vi "未命名 3.vi"() -> ()   [LabVIEW 2018]
panel:
  in  "数值":dbl
  out "簇 2":cluster{"数值":dbl, "数值 2":dbl}
  in  "簇":cluster{"数值":dbl, "数值 2":dbl}
  out "数组 3":i32[][](array[numeric])
  out "添加的数组":dbl[](array[numeric])
  out "数组 2":i32[](array[numeric])
  in  "数组":dbl[](array[numeric])
  out "波形图 2":dynamicdata(graph)
  out "波形图":dynamicdata(graph)
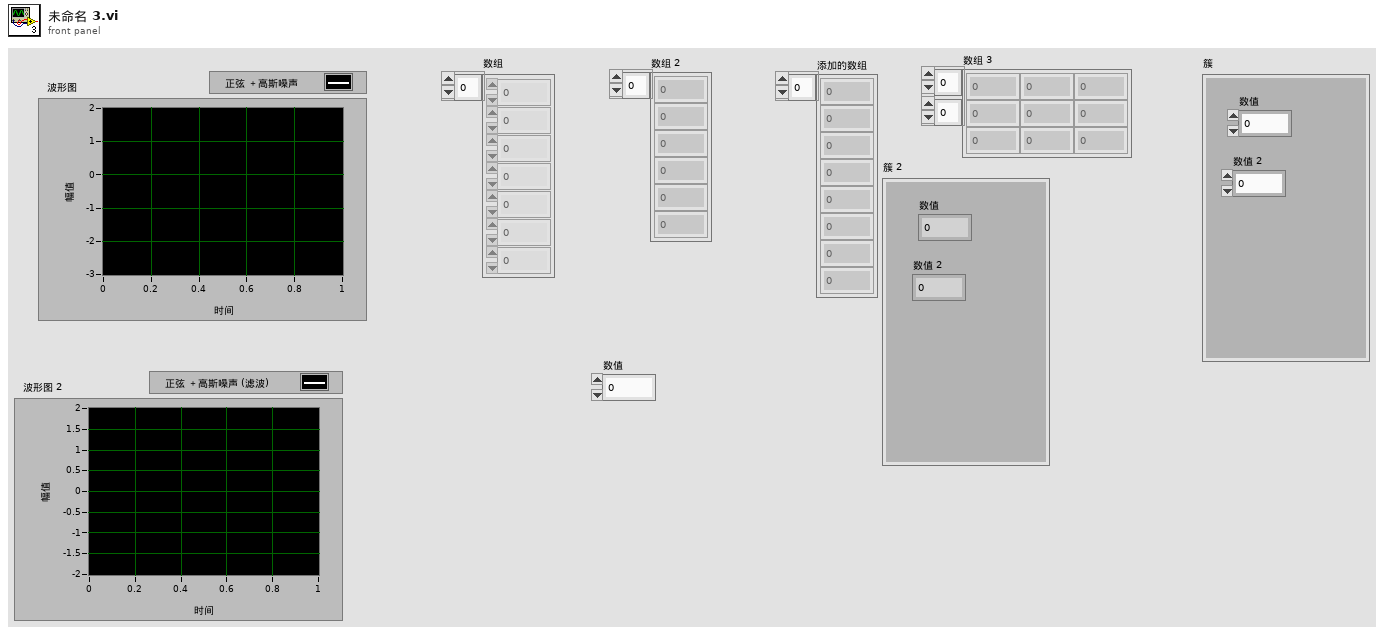
[diagram p1: front panel]
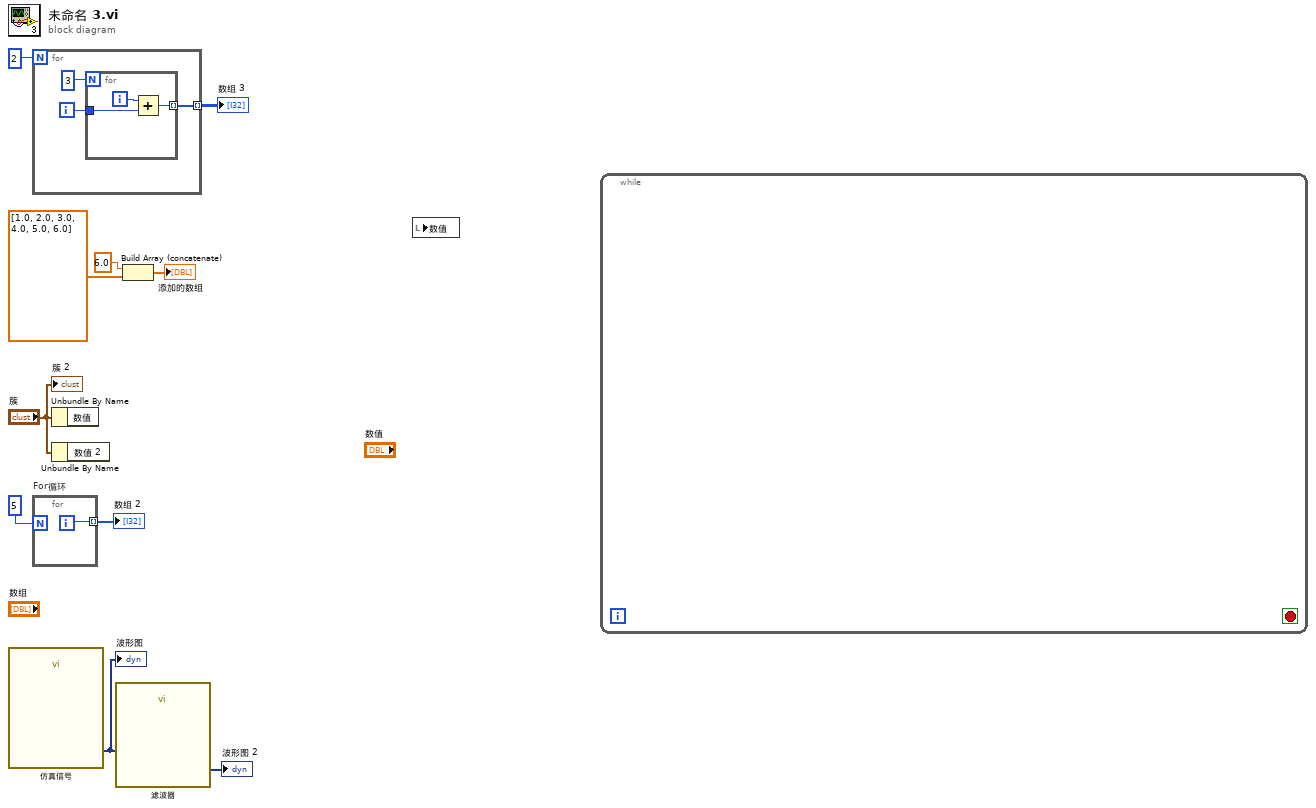
[diagram p0: block diagram]
diagram:
  n1 = call "仿真信号"() -> ("正弦与高斯噪声"=w10:dynamicdata)  [unwired: 14 in, 1 out]
  "波形图" <- w10
  n2 = for {
    N: 2 -> [_]
    tunnel: [w11] -> w2 mode=indexing
    i -> [w12]
    n3 = for {
      N: 3 -> [_]
      tunnel: w12 -> [w16]
      tunnel: [w14] -> w11 mode=indexing
      i -> [w15]
      n4 = Add(x=w15, y=w16) -> (x+y=w14:i32)
    }
  }
  "数组 3" <- w2
  n5 = for "For循环" {
    N: 5 -> [_]
    tunnel: [w17] -> w7 mode=indexing
    i -> [w17]
  }
  "数组 2" <- w7
  n6 = Unbundle By Name("簇") -> ()  [unwired: 1 out]
  n7 = Unbundle By Name("簇") -> ()  [unwired: 1 out]
  n8 = call "滤波器"("Signal"=w10) -> ("Filtered Signal"=→"波形图 2":dynamicdata)  [unwired: 9 in, 1 out]
  n9 = Build Array (concatenate)(6.0 ("数组"), dbl[] [1.0, 2.0, 3.0, 4.0, 5.0, 6.0] ("数组")) -> (→"添加的数组":dbl[])
  n10 = local read "数值"() -> ()  [unwired: 1 in]
  n11 = while {
    stop <- _ stop-if-true
  }
  "簇 2" <- "簇"
